vi "Calculate Window Bounds.vi"(6 "Horizontal Alignment":T3, 8 "error in (no error)":errorcluster, 9 "Vertical Alignment":T2, 10 "Position (Screen)":T1, 11 "VI in":refnum<vi>) -> (0 "error out":errorcluster, 2 "Front Panel Window:Window Bounds":T4, 3 "VI out":refnum<vi>)   [LabVIEW 2012, in "Win8uiDemo.lvlib" / "Flyout.lvclass"]
uses:
  Flyout.lvclass
  <vilib>/Utility/miscctls.llb/LVRectTypeDef.ctl
  Horizontal Alignment.ctl
  Vertical Alignment.ctl
  <vilib>/Utility/miscctls.llb/LVPositionTypeDef.ctl
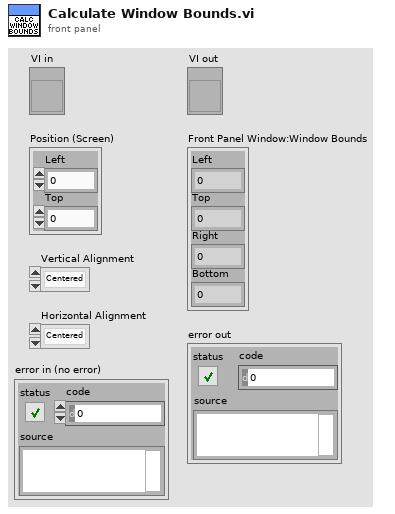
[diagram p1: front panel]
types:
  T1 = typedef "LVPositionTypeDef.ctl" = cluster{"Left":i32, "Top":i32}
  T2 = typedef "Win8uiDemo.lvlib/Flyout.lvclass/Vertical Alignment.ctl" = enum16{"Centered", "Above", "Below"}
  T3 = typedef "Win8uiDemo.lvlib/Flyout.lvclass/Horizontal Alignment.ctl" = enum16{"Centered", "Left", "Right"}
  T4 = typedef "LVRectTypeDef.ctl" = cluster{"Left":i16, "Top":i16, "Right":i16, "Bottom":i16}
  T5 = enum32{"Invalid", "Standard", "Closed", "Hidden", "Minimized", "Maximized"}
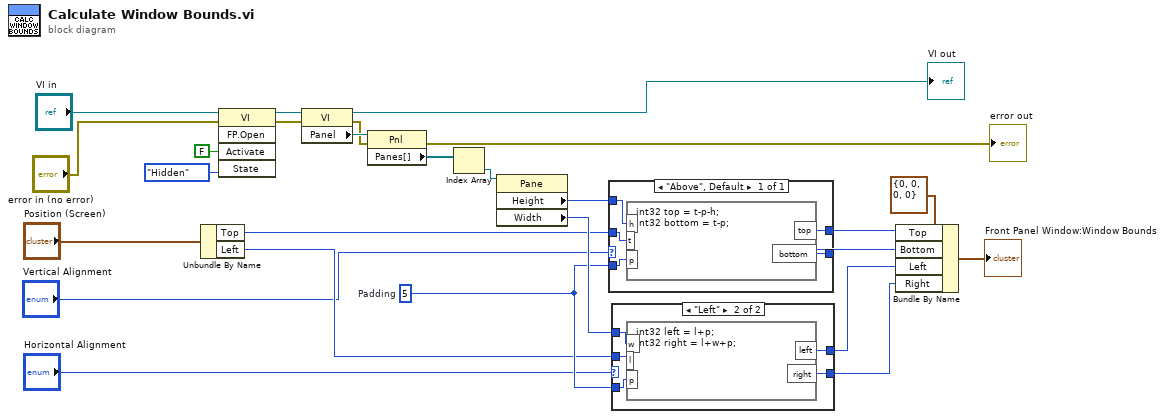
[diagram p0: block diagram]
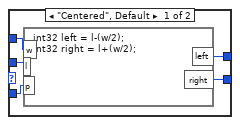
[diagram p2: hidden frame]
diagram:
  w12 = 5  # Padding
  n1 = Unbundle By Name("Position (Screen)") -> ("Top"=w8:i32, "Left"=w11:i32)
  n2 = invoke class="VI" method="FP.Open"(reference="VI in", error in="error in (no error)", "Activate"=FALSE ("Activate?"), "State"=T5."Hidden") -> (reference out=w4:refnum<vi>, error out=w5:errorcluster)  [unwired: 1 in, 3 out]
  n3 = property class="VI"(reference=w4, error in=w5) -> (reference out=→"VI out":refnum<vi>, error out=w6:errorcluster, "Panel"=w22:refnum<vi>)
  n4 = property class="Pnl"(reference=w22, error in=w6) -> (error out=→"error out":errorcluster, "Panes[]"=w25:refnum<vi>[])  [unwired: 1 out]
  n5 = Index Array(array=w25) -> (element=w26:refnum<vi>)  [unwired: 1 in]
  n6 = property class="Pane"(reference=w26) -> ("Height"=w23:u32, "Width"=w24:u32)  [unwired: 1 in, 2 out]
  n7 = case shown="\"Above\", Default" "Vertical Alignment" {
    tunnel: w23 -> [w31]
    tunnel: w8 -> [w30]
    tunnel: w12 -> [w29]
    tunnel: [w28] -> w18
    tunnel: [w27] -> w19
    frame "Above", Default {
      n8 = formula code="int32 top = t-p-h;\nint32 bottom = t-p;"("h"=w31, "t"=w30, "p"=w29) -> ("top"=w28:i32, "bottom"=w27:i32)
    }
  }
  n9 = case shown="\"Left\"" "Horizontal Alignment" {
    tunnel: w24 -> [w34 w39]
    tunnel: w11 -> [w36 w41]
    tunnel: w12 -> [w35 w40]
    tunnel: [w33 w38] -> w20
    tunnel: [w32 w37] -> w21
    frame "Centered", Default {
      n10 = formula code="int32 left = l-(w/2);\nint32 right = l+(w/2);"("w"=w34, "l"=w36, "p"=w35) -> ("left"=w33:i32, "right"=w32:i32)
    }
    frame "Left" {
      n11 = formula code="int32 left = l+p;\nint32 right = l+w+p;"("w"=w39, "l"=w41, "p"=w40) -> ("left"=w38:i32, "right"=w37:i32)
    }
  }
  n12 = Bundle By Name(cluster=T4 {"Left"=0, "Top"=0, "Right"=0, "Bottom"=0} ("Front Panel Window:Window Bounds"), "Top"=w18, "Bottom"=w19, "Left"=w20, "Right"=w21) -> (→"Front Panel Window:Window Bounds":T4)
